vi "2_AdvancedDemo_MHHisto.vi"() -> ()   [LabVIEW 2010]
uses:
  Types/MH_UIThread_Cmds.ctl
  _lib/PQ/MultiHarp/MH_InitInfo.ctl
  Types/MH_UIThread_Data.ctl
  Types/MH_InputChannel.ctl
  _lib/PQ/MultiHarp/MH_RefSource.ctl
  _lib/PQ/MultiHarp/mhlib_x86_x64_UIThread.llb/MH_DllPath_global.vi
  <vilib>/Utility/error.llb/DialogType.ctl
  _lib/PQ/MultiHarp/MH_LibVersion_global.vi
  _lib/PQ/MultiHarp/MH_MeasMode.ctl
  Types/MH_SetInpChanData.ctl
  Types/MH_SetInpChanCmds.ctl
panel:
  in  "Settings":bool=TRUE
  in  "Run continuously":bool=TRUE caption="Conti."
  in  "Start":bool
  in  "Scale":bool
  out "CountRates":i32[](graph)
  in  "AllChannels":T1={"Enable"=TRUE, "Offset"=0, "Level"=-100, "Edge"=0, "DeadTime"=1000, "UseDeadTime"=FALSE, "SetEnableAllChan"=TRUE, "SetEdgeAllChan"=TRUE, "SetLevelAllChan"=TRUE, "SetOffsetAllChan"=TRUE, "SetUseDTAllChan"=TRUE, "SetDeadTAllChan"=TRUE} {"DeadTime" min=800 max=160000 step=1; "Edge" items=["falling", "rising"]; "Offset" min=-100000 max=100000 step=5; "Level" min=-1200 max=1200 step=1}
  in  "HistoLength":i32(ring)=6 caption="Num Bins" items=["1024", "2048", "4096", "8192", "16384", "32768", "65536"]
  in  "OvlLevel":u32=4294967295 caption="Ovl.Level" min=1 step=1
  in  "StopOvl.":bool=TRUE
  in  "AcqTime":i32=1000 caption="Acqu.           ms" min=1 max=360000 step=1
  in  "Binning":i32(ring) caption="Resol.            ps" items=["5", "10", "20", "40", "80", "160", "320", "640", "1280", "2560", "5120", "10240", "20480", "40960", "81920", "163840", "327680", "655360", "1310720", "2621440", "5242880", "10485760", "20971520", "41943040"]
  in  "HistoOffset":i32 caption="Offset            ns" min=0 max=100000000 step=1
  out "HistoGraph":T2(graph)={0.0, "Resolution"=0.005, "Histogram"=array64x1024[65536 elements]}
  in  "SyncDeadTime":i32=1000 caption="Dead T.   ps" min=800 max=160000 step=1
  in  "UseDeadTime":bool caption="Use DT."
  in  "SyncEdge":i32(ring) caption="Edge" items=["falling", "rising"]
  in  "SyncDivider":i32(ring) caption="Divider" items=["1", "2", "4", "8", "16"]
  in  "SyncOffset":i32 caption="Offset      ps" min=-100000 max=100000 step=5
  in  "SyncLevel":i32=-100 caption="Level      mV" min=-1200 max=1200 step=1
  in  "Channels":T3[](array[typedef])=[{"Name"="Inp.Chan 1", "Enable"=TRUE, "Edge"=0, "Level"=-100, "Offset"=0, "UseDeadTime"=FALSE, "DeadTime"=1000}, {"Name"="Inp.Chan 2", "Enable"=TRUE, "Edge"=0, "Level"=-100, "Offset"=0, "UseDeadTime"=FALSE, "DeadTime"=1000}, {"Name"="Inp.Chan 3", "Enable"=TRUE, "Edge"=0, "Level"=-100, "Offset"=0, "UseDeadTime"=FALSE, "DeadTime"=1000}, {"Name"="Inp.Chan 4", "Enable"=TRUE, "Edge"=0, "Level"=-100, "Offset"=0, "UseDeadTime"=FALSE, "DeadTime"=1000}, {"Name"="Inp.Chan 5", "Enable"=TRUE, "Edge"=0, "Level"=-100, "Offset"=0, "UseDeadTime"=FALSE, "DeadTime"=1000}, {"Name"="Inp.Chan 6", "Enable"=TRUE, "Edge"=0, "Level"=-100, "Offset"=0, "UseDeadTime"=FALSE, "DeadTime"=1000}, {"Name"="Inp.Chan 7", "Enable"=TRUE, "Edge"=0, "Level"=-100, "Offset"=0, "UseDeadTime"=FALSE, "DeadTime"=1000}, {"Name"="Inp.Chan 8", "Enable"=TRUE, "Edge"=0, "Level"=-100, "Offset"=0, "UseDeadTime"=FALSE, "DeadTime"=1000}, {"Name"="Inp.Chan 9", "Enable"=TRUE, "Edge"=0, "Level"=-100, "Offset"=0, "UseDeadTime"=FALSE, "DeadTime"=1000}, {"Name"="Inp.Chan 10", "Enable"=TRUE, "Edge"=0, "Level"=-100, "Offset"=0, "UseDeadTime"=FALSE, "DeadTime"=1000}, {"Name"="Inp.Chan 11", "Enable"=TRUE, "Edge"=0, "Level"=-100, "Offset"=0, "UseDeadTime"=FALSE, "DeadTime"=1000}, {"Name"="Inp.Chan 12", "Enable"=TRUE, "Edge"=0, "Level"=-100, "Offset"=0, "UseDeadTime"=FALSE, "DeadTime"=1000}, {"Name"="Inp.Chan 13", "Enable"=TRUE, "Edge"=0, "Level"=-100, "Offset"=0, "UseDeadTime"=FALSE, "DeadTime"=1000}, {"Name"="Inp.Chan 14", "Enable"=TRUE, "Edge"=0, "Level"=-100, "Offset"=0, "UseDeadTime"=FALSE, "DeadTime"=1000}, {"Name"="Inp.Chan 15", "Enable"=TRUE, "Edge"=0, "Level"=-100, "Offset"=0, "UseDeadTime"=FALSE, "DeadTime"=1000}, {"Name"="Inp.Chan 16", "Enable"=TRUE, "Edge"=0, "Level"=-100, "Offset"=0, "UseDeadTime"=FALSE, "DeadTime"=1000}, {"Name"="Inp.Chan 17", "Enable"=TRUE, "Edge"=0, "Level"=-100, "Offset"=0, "UseDeadTime"=FALSE, "DeadTime"=1000}, {"Name"="Inp.Chan 18", "Enable"=TRUE, "Edge"=0, "Level"=-100, "Offset"=0, "UseDeadTime"=FALSE, "DeadTime"=1000}, {"Name"="Inp.Chan 19", "Enable"=TRUE, "Edge"=0, "Level"=-100, "Offset"=0, "UseDeadTime"=FALSE, "DeadTime"=1000}, {"Name"="Inp.Chan 20", "Enable"=TRUE, "Edge"=0, "Level"=-100, "Offset"=0, "UseDeadTime"=FALSE, "DeadTime"=1000}, {"Name"="Inp.Chan 21", "Enable"=TRUE, "Edge"=0, "Level"=-100, "Offset"=0, "UseDeadTime"=FALSE, "DeadTime"=1000}, {"Name"="Inp.Chan 22", "Enable"=TRUE, "Edge"=0, "Level"=-100, "Offset"=0, "UseDeadTime"=FALSE, "DeadTime"=1000}, {"Name"="Inp.Chan 23", "Enable"=TRUE, "Edge"=0, "Level"=-100, "Offset"=0, "UseDeadTime"=FALSE, "DeadTime"=1000}, {"Name"="Inp.Chan 24", "Enable"=TRUE, "Edge"=0, "Level"=-100, "Offset"=0, "UseDeadTime"=FALSE, "DeadTime"=1000}, {"Name"="Inp.Chan 25", "Enable"=TRUE, "Edge"=0, "Level"=-100, "Offset"=0, "UseDeadTime"=FALSE, "DeadTime"=1000}, {"Name"="Inp.Chan 26", "Enable"=TRUE, "Edge"=0, "Level"=-100, "Offset"=0, "UseDeadTime"=FALSE, "DeadTime"=1000}, {"Name"="Inp.Chan 27", "Enable"=TRUE, "Edge"=0, "Level"=-100, "Offset"=0, "UseDeadTime"=FALSE, "DeadTime"=1000}, {"Name"="Inp.Chan 28", "Enable"=TRUE, "Edge"=0, "Level"=-100, "Offset"=0, "UseDeadTime"=FALSE, "DeadTime"=1000}, {"Name"="Inp.Chan 29", "Enable"=TRUE, "Edge"=0, "Level"=-100, "Offset"=0, "UseDeadTime"=FALSE, "DeadTime"=1000}, {"Name"="Inp.Chan 30", "Enable"=TRUE, "Edge"=0, "Level"=-100, "Offset"=0, "UseDeadTime"=FALSE, "DeadTime"=1000}, {"Name"="Inp.Chan 31", "Enable"=TRUE, "Edge"=0, "Level"=-100, "Offset"=0, "UseDeadTime"=FALSE, "DeadTime"=1000}, {"Name"="Inp.Chan 32", "Enable"=TRUE, "Edge"=0, "Level"=-100, "Offset"=0, "UseDeadTime"=FALSE, "DeadTime"=1000}, {"Name"="Inp.Chan 33", "Enable"=TRUE, "Edge"=0, "Level"=-100, "Offset"=0, "UseDeadTime"=FALSE, "DeadTime"=1000}, {"Name"="Inp.Chan 34", "Enable"=TRUE, "Edge"=0, "Level"=-100, "Offset"=0, "UseDeadTime"=FALSE, "DeadTime"=1000}, {"Name"="Inp.Chan 35", "Enable"=TRUE, "Edge"=0, "Level"=-100, "Offset"=0, "UseDeadTime"=FALSE, "DeadTime"=1000}, {"Name"="Inp.Chan 36", "Enable"=TRUE, "Edge"=0, "Level"=-100, "Offset"=0, "UseDeadTime"=FALSE, "DeadTime"=1000}, {"Name"="Inp.Chan 37", "Enable"=TRUE, "Edge"=0, "Level"=-100, "Offset"=0, "UseDeadTime"=FALSE, "DeadTime"=1000}, {"Name"="Inp.Chan 38", "Enable"=TRUE, "Edge"=0, "Level"=-100, "Offset"=0, "UseDeadTime"=FALSE, "DeadTime"=1000}, {"Name"="Inp.Chan 39", "Enable"=TRUE, "Edge"=0, "Level"=-100, "Offset"=0, "UseDeadTime"=FALSE, "DeadTime"=1000}, {"Name"="Inp.Chan 40", "Enable"=TRUE, "Edge"=0, "Level"=-100, "Offset"=0, "UseDeadTime"=FALSE, "DeadTime"=1000}, {"Name"="Inp.Chan 41", "Enable"=TRUE, "Edge"=0, "Level"=-100, "Offset"=0, "UseDeadTime"=FALSE, "DeadTime"=1000}, {"Name"="Inp.Chan 42", "Enable"=TRUE, "Edge"=0, "Level"=-100, "Offset"=0, "UseDeadTime"=FALSE, "DeadTime"=1000}, {"Name"="Inp.Chan 43", "Enable"=TRUE, "Edge"=0, "Level"=-100, "Offset"=0, "UseDeadTime"=FALSE, "DeadTime"=1000}, {"Name"="Inp.Chan 44", "Enable"=TRUE, "Edge"=0, "Level"=-100, "Offset"=0, "UseDeadTime"=FALSE, "DeadTime"=1000}, {"Name"="Inp.Chan 45", "Enable"=TRUE, "Edge"=0, "Level"=-100, "Offset"=0, "UseDeadTime"=FALSE, "DeadTime"=1000}, {"Name"="Inp.Chan 46", "Enable"=TRUE, "Edge"=0, "Level"=-100, "Offset"=0, "UseDeadTime"=FALSE, "DeadTime"=1000}, {"Name"="Inp.Chan 47", "Enable"=TRUE, "Edge"=0, "Level"=-100, "Offset"=0, "UseDeadTime"=FALSE, "DeadTime"=1000}, {"Name"="Inp.Chan 48", "Enable"=TRUE, "Edge"=0, "Level"=-100, "Offset"=0, "UseDeadTime"=FALSE, "DeadTime"=1000}, {"Name"="Inp.Chan 49", "Enable"=TRUE, "Edge"=0, "Level"=-100, "Offset"=0, "UseDeadTime"=FALSE, "DeadTime"=1000}, {"Name"="Inp.Chan 50", "Enable"=TRUE, "Edge"=0, "Level"=-100, "Offset"=0, "UseDeadTime"=FALSE, "DeadTime"=1000}, {"Name"="Inp.Chan 51", "Enable"=TRUE, "Edge"=0, "Level"=-100, "Offset"=0, "UseDeadTime"=FALSE, "DeadTime"=1000}, {"Name"="Inp.Chan 52", "Enable"=TRUE, "Edge"=0, "Level"=-100, "Offset"=0, "UseDeadTime"=FALSE, "DeadTime"=1000}, {"Name"="Inp.Chan 53", "Enable"=TRUE, "Edge"=0, "Level"=-100, "Offset"=0, "UseDeadTime"=FALSE, "DeadTime"=1000}, {"Name"="Inp.Chan 54", "Enable"=TRUE, "Edge"=0, "Level"=-100, "Offset"=0, "UseDeadTime"=FALSE, "DeadTime"=1000}, {"Name"="Inp.Chan 55", "Enable"=TRUE, "Edge"=0, "Level"=-100, "Offset"=0, "UseDeadTime"=FALSE, "DeadTime"=1000}, {"Name"="Inp.Chan 56", "Enable"=TRUE, "Edge"=0, "Level"=-100, "Offset"=0, "UseDeadTime"=FALSE, "DeadTime"=1000}, {"Name"="Inp.Chan 57", "Enable"=TRUE, "Edge"=0, "Level"=-100, "Offset"=0, "UseDeadTime"=FALSE, "DeadTime"=1000}, {"Name"="Inp.Chan 58", "Enable"=TRUE, "Edge"=0, "Level"=-100, "Offset"=0, "UseDeadTime"=FALSE, "DeadTime"=1000}, {"Name"="Inp.Chan 59", "Enable"=TRUE, "Edge"=0, "Level"=-100, "Offset"=0, "UseDeadTime"=FALSE, "DeadTime"=1000}, {"Name"="Inp.Chan 60", "Enable"=TRUE, "Edge"=0, "Level"=-100, "Offset"=0, "UseDeadTime"=FALSE, "DeadTime"=1000}, {"Name"="Inp.Chan 61", "Enable"=TRUE, "Edge"=0, "Level"=-100, "Offset"=0, "UseDeadTime"=FALSE, "DeadTime"=1000}, {"Name"="Inp.Chan 62", "Enable"=TRUE, "Edge"=0, "Level"=-100, "Offset"=0, "UseDeadTime"=FALSE, "DeadTime"=1000}, {"Name"="Inp.Chan 63", "Enable"=TRUE, "Edge"=0, "Level"=-100, "Offset"=0, "UseDeadTime"=FALSE, "DeadTime"=1000}, {"Name"="Inp.Chan 64", "Enable"=TRUE, "Edge"=0, "Level"=-100, "Offset"=0, "UseDeadTime"=FALSE, "DeadTime"=1000}] {"DeadTime" min=800 max=160000 step=1; "Edge" items=["falling", "rising"]; "Offset" min=-100000 max=100000 step=5; "Level" min=-1200 max=1200 step=1}
  out "SyncRate":string="Sync Rate: 0 cps\n"
  out "OverFlow":bool caption="Overflow:"
  out "Status":string="Initialized!"
  # "Acquisition"
  # "All Channels"
  # "Sync"
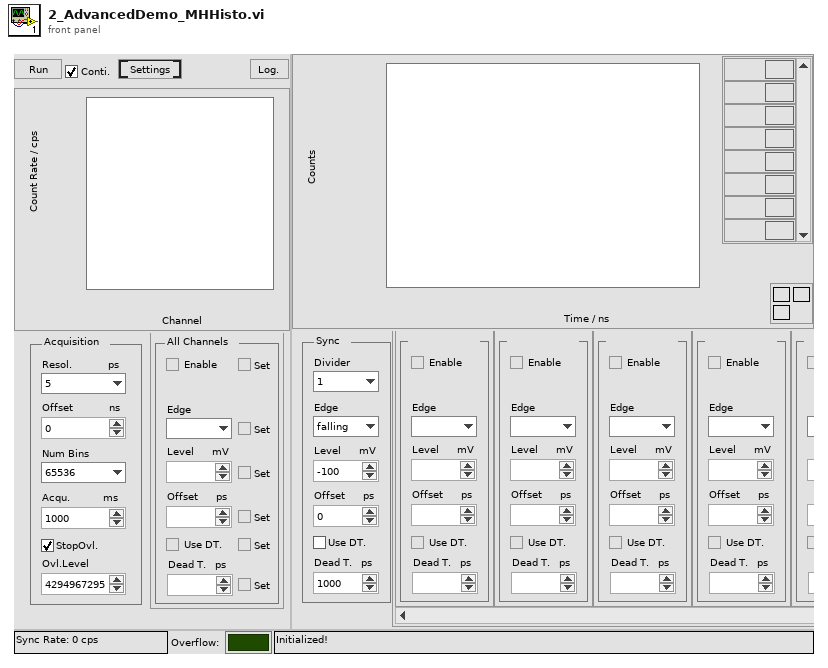
[diagram p1: front panel]
types:
  T1 = cluster{"Enable":bool, "Offset":i32, "Level":i32, "Edge":i32, "DeadTime":i32, "UseDeadTime":bool, "SetEnableAllChan":bool, "SetEdgeAllChan":bool, "SetLevelAllChan":bool, "SetOffsetAllChan":bool, "SetUseDTAllChan":bool, "SetDeadTAllChan":bool}
  T2 = cluster{dbl, "Resolution":dbl, "Histogram":u32[][]}
  T3 = typedef "MH_InputChannel.ctl" = cluster{"Name":string, "Enable":bool, "Edge":i32, "Level":i32, "Offset":i32, "UseDeadTime":bool, "DeadTime":i32}
  T4 = typedef "MH_UIThread_Data.ctl" = cluster{"Init Info":T5, "DevIdx":i32, "SyncDivider":i32, "SyncOffset":i32, "SyncLevel":i32, "Channels":T3[], "CurrentChannels":i32[], "AcqTime":i32, "Binning":i32, "HistoOffset":i32, "HistoLen":i32, "StopOvl.":bool, "OvlLevel":u32, "SyncEdge":i32, "StartMeas":bool, "HistoLength":i32, "Resolution":dbl, "Run cont.":bool, "Status":string, "SyncRate":i32, "BitShift":i32, "HistoAcqTime":dbl, "SyncRateStart":i32, "UseDeadTime":bool, "SyncDeadTime":i32, "SetInpChan":T6[]}
  T5 = typedef "MH_InitInfo.ctl" = cluster{"Library Version":string, "Serial No.":string, "Model":string, "Partnum":string, "Version":string, "features":i32, "nchannels":i32, "Base Resolution":dbl, "Bin Steps":i32}
  T6 = typedef "MH_SetInpChanData.ctl" = cluster{"Channel":i32, "Cmds":T7[], "Changed":cluster{"Name":bool, "Enable":bool, "Edge":bool, "Level":bool, "Offset":bool, "UseDeadTime":bool, "DeadTime":bool}}
  T7 = typedef "MH_SetInpChanCmds.ctl" = enum16{"SetInpChanEnable", "SetInpChanOffset", "SetInpChanDeadTime", "SetInpChanTrg"}
  T8 = typedef "MH_UIThread_Cmds.ctl" = enum16{"Idle", "Init", "SetInpChan", "SetSyncDivider", "SetSyncTrg", "SetSyncOffset", "SetSyncDeadTime", "SetBinning", "SetHistoOffset", "SetHistoLen", "SetStopOvl", "SetBitShift", "SetHistoAcqTime", "GetRates", "GetAllRates", "StartMeas", "StopMeas", "AbortMeas", "GetResolution", "GetHistos", "GetAllHistos", "ReadFiFo", "WriteStatus", "Resize", "EnableControls", "DisableControls", "Error", "Exit"}
  T9 = enum8{"Enabled", "Disabled", "Disabled and Grayed Out"}
  T10 = cluster{"[0]":bool, "[1]":bool, "[2]":bool, "[3]":bool, "[4]":bool, "[5]":bool}
  T11 = typedef "MH_MeasMode.ctl" = i32
  T12 = typedef "MH_RefSource.ctl" = enum16{"INTERNAL", "EXTERNAL_10MHZ", "WR_MASTER_GENERIC", "WR_SLAVE_GENERIC", "WR_GRANDM_GENERIC", "EXTN_GPS_PPS", "EXTN_GPS_PPS_UART", "WR_MASTER_MHARP", "WR_SLAVE_MHARP", "WR_GRANDM_MHARP"}
  T13 = cluster{dbl, "Resolution":dbl, "Histograms":u32[][]}
  T14 = typedef "DialogType.ctl" = u16
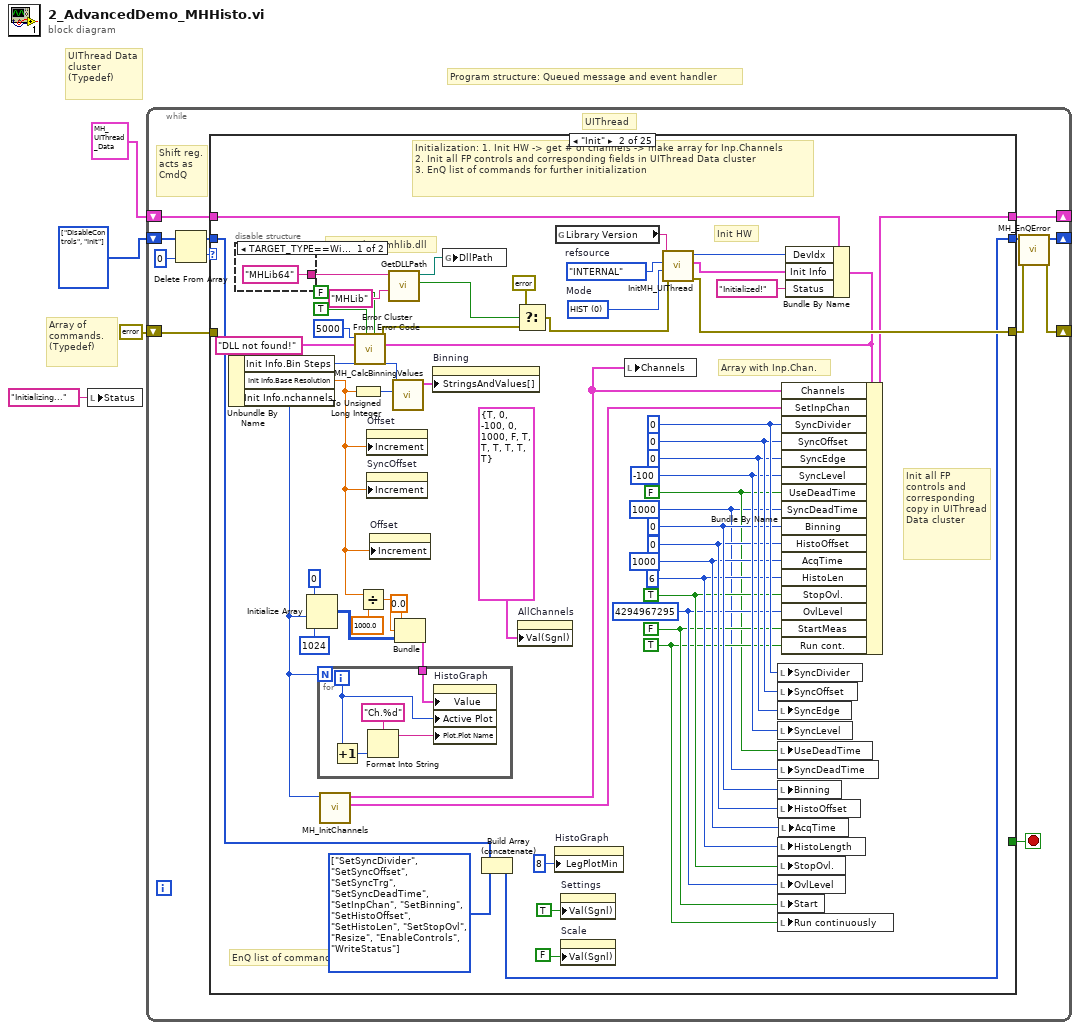
[diagram p0: block diagram]
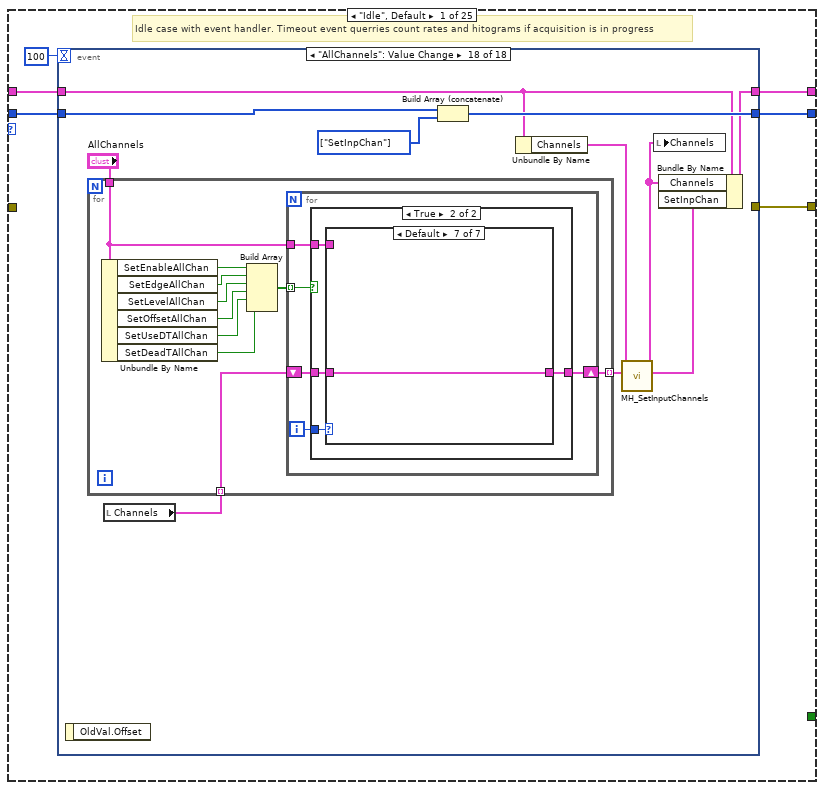
[diagram p2: hidden frame]
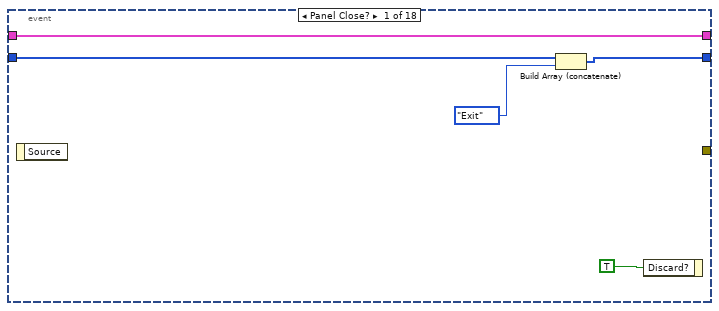
[diagram p3: hidden frame]
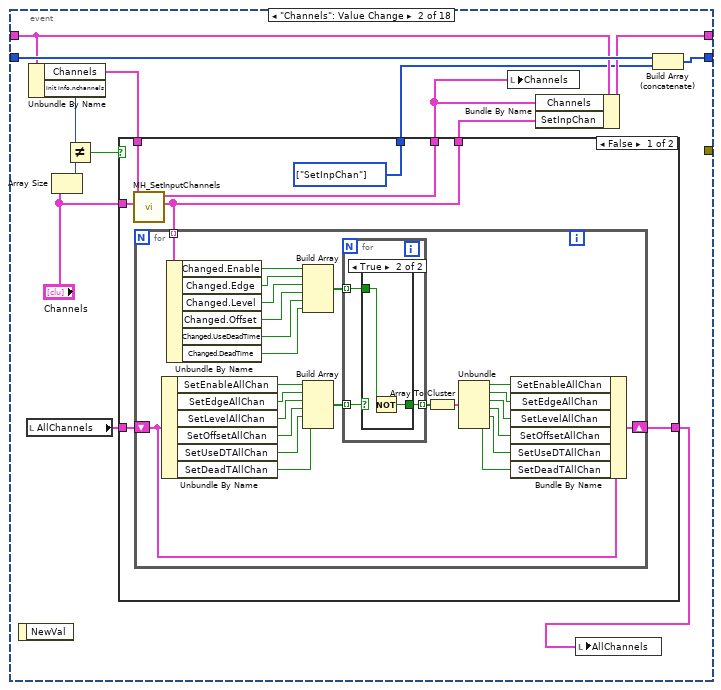
[diagram p4: hidden frame]
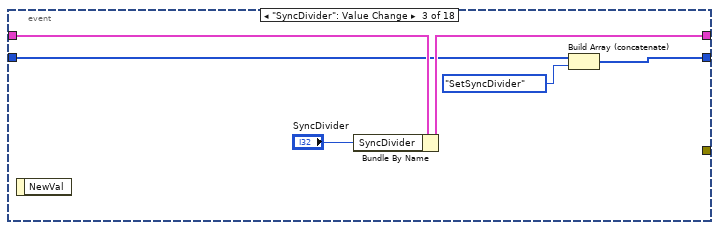
[diagram p7: hidden frame]
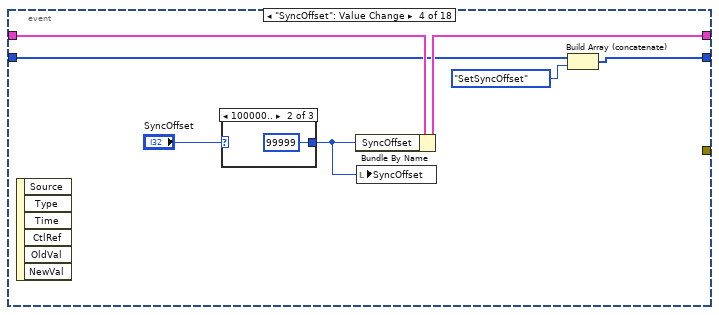
[diagram p8: hidden frame]
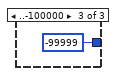
[diagram p10: hidden frame]
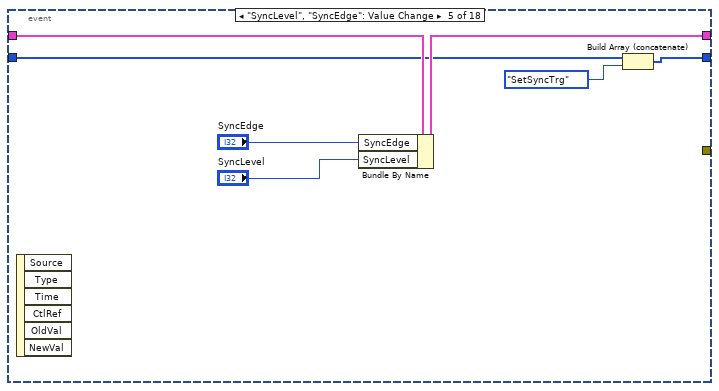
[diagram p11: hidden frame]
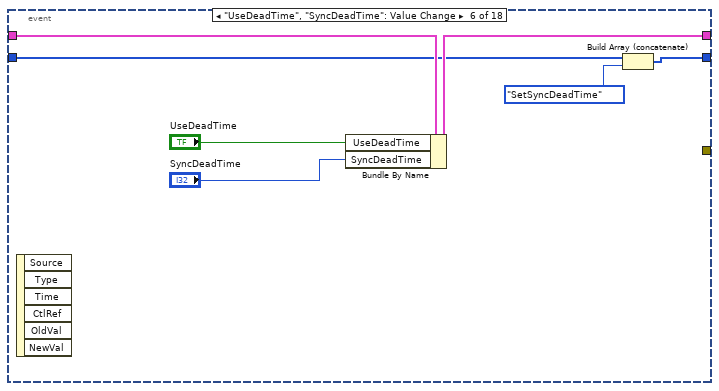
[diagram p12: hidden frame]
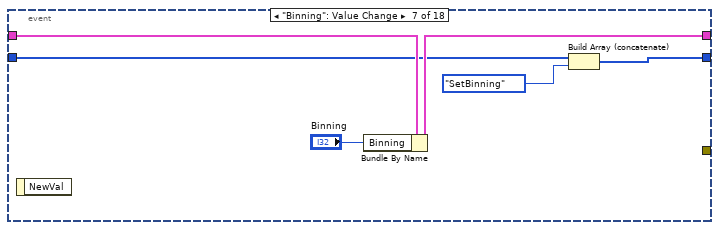
[diagram p13: hidden frame]
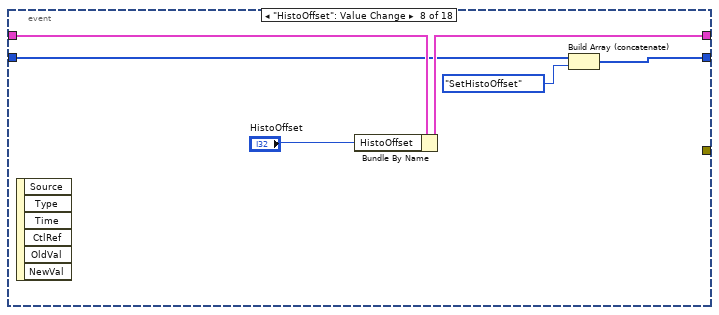
[diagram p14: hidden frame]
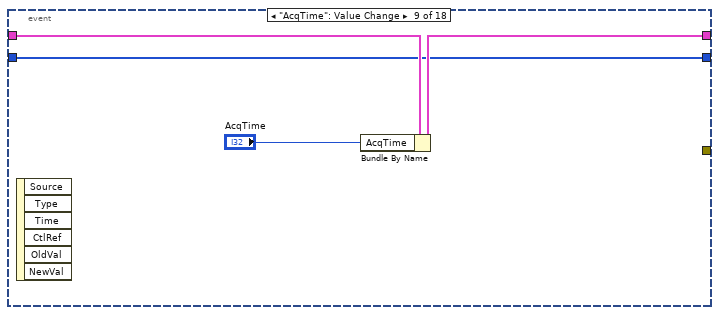
[diagram p15: hidden frame]
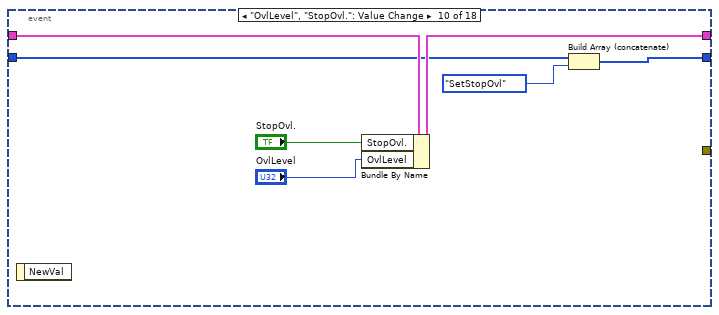
[diagram p16: hidden frame]
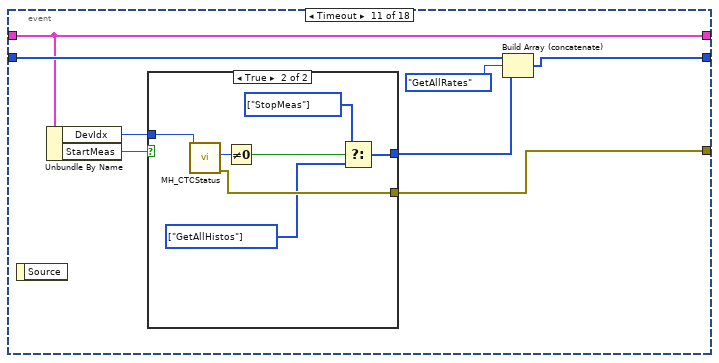
[diagram p17: hidden frame]
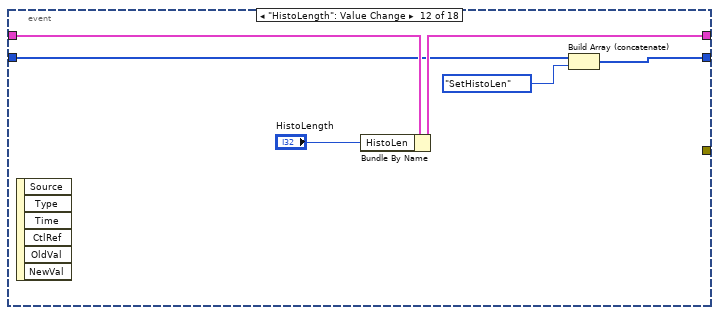
[diagram p19: hidden frame]
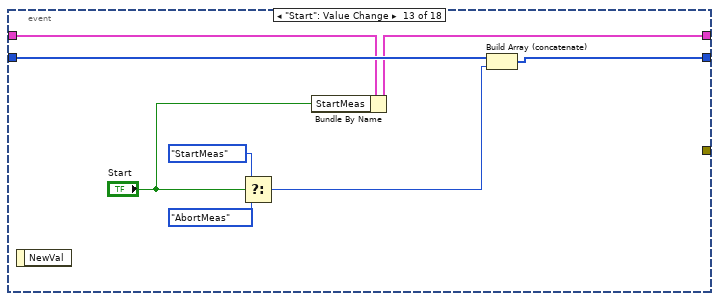
[diagram p20: hidden frame]
diagram:
  w3 = T8[] [enum."DisableControls", enum."Init"] items=["Idle", "Init", "SetInpChan", "SetSyncDivider", "SetSyncTrg", "SetSyncOffset", "SetSyncDeadTime", "SetBinning", "SetHistoOffset", "SetHistoLen", "SetStopOvl", "SetBitShift", "SetHistoAcqTime", "GetRates", "GetAllRates", "StartMeas", "StopMeas", "AbortMeas", "GetResolution", "GetHistos", "GetAllHistos", "ReadFiFo", "WriteStatus", "Resize", "EnableControls", "DisableControls", "Error", "Exit"]
  # "Array of commands.\n(Typedef)"
  # "Program structure: Queued message and event handler"
  # "UIThread Data cluster\n(Typedef)"
  n1 = local write "Status"("Initializing..." ("Status")) -> ()
  n2 = while {
    shift-right: [w5] -> _
    shift-left: w3 -> [w12]
    shift-right: [w15] -> _
    shift-left: T4 {"Init Info"={"Library Version"="", "Serial No."="", "Model"="", "Partnum"="", "Version"="", "features"=0, "nchannels"=0, "Base Resolution"=0.0, "Bin Steps"=0}, "DevIdx"=0, "SyncDivider"=1, "SyncOffset"=0, "SyncLevel"=50, "Channels"=[], "CurrentChannels"=[], "AcqTime"=1, "Binning"=1, "HistoOffset"=1, "HistoLen"=1024, "StopOvl."=FALSE, "OvlLevel"=1024, "SyncEdge"=10, "StartMeas"=FALSE, "HistoLength"=0, "Resolution"=0.0, "Run cont."=FALSE, "Status"="", "SyncRate"=0, "BitShift"=0, "HistoAcqTime"=0.0, "SyncRateStart"=0, "UseDeadTime"=FALSE, "SyncDeadTime"=800, "SetInpChan"=[]} -> [w14]
    shift-right: [w7] -> _
    shift-left: errorcluster {"status"=FALSE, "code"=0, "source"=""} ("error IO") -> [w13]
    stop <- w16 stop-if-true
    # "Shift reg.\nacts as\nCmdQ"
    # "UIThread"
    n3 = Delete From Array(array=w12, index=0) -> (deleted portion=w10:T8, array with subset deleted=w9:T8[])  [unwired: 1 in]
    n4 = case shown="\"Init\"" w10 {
      tunnel: [w22 w305 w324 w386 w395 w407 w413 w420 w428 w436 w441 w452 w463 w478 w486 w500 w514 w539 w571 w595 w608 w615 w627 w633 w637] -> w6
      tunnel: [_ _ _ _ _ _ _ _ _ _ _ _ _ _ _ _ _ _ _ _ _ _ _ _ TRUE] -> w16
      tunnel: [w21 w285 w325 w388 w396 w408 w417 w424 w429 w431 w442 w451 w462 w484 w489 w503 w510 w538 w570 w594 w596 w614 w626 w634 w640] -> w15
      tunnel: w14 -> [w20 w290 w325 w388 w396 w408 w417 w424 w429 w432 w442 w451 w462 w484 w490 w504 w511 w538 w570 w594 w596 w614 w626 w634 w640]
      tunnel: [w17 w308 w322 w384 w394 w406 w416 w423 w427 w435 w440 w445 w461 w483 w492 w506 w512 w536 w566 _ _ _ _ _ w638] -> w8
      tunnel: w13 -> [_ _ _ _ _ _ _ _ _ _ _ _ _ _ _ _ _ _ _ _ _ _ _ w635 _]
      tunnel: w9 -> [w19 w307 w324 w386 w395 w407 w413 w419 w428 w436 w441 w452 w463 w479 w487 w501 w514 w539 w571 w595 w608 w615 w627 _ w637]
      frame "Idle", Default {
        # "Idle case with event handler. Timeout event querries count rates and hitograms if acquisition is in progress"
        n5 = event shown="[17] \"AllChannels\": Value Change" {
          selector: _ -> [_ _ _ _ _ _ _ _ _ _ _ _ _ _ _ _ _ _]
          dyn-events: _ -> [_ _ _ _ _ _ _ _ _ _ _ _ _ _ _ _ _ _]
          timeout: 100 -> [_ _ _ _ _ _ _ _ _ _ _ _ _ _ _ _ _ _]
          tunnel: [w23 w40 w82 w90 w99 w107 w113 w119 w124 w130 w140 w151 w159 w167 w173 w181 w191 w204] -> w22
          tunnel: [w26 w33 w86 w93 w103 w110 w116 w122 w126 w133 w139 w154 w157 w165 w172 w180 w194 w198] -> w21
          tunnel: w20 -> [w26 w35 w87 w94 w104 w111 w117 w123 w127 w134 w139 w155 w158 w166 w172 w180 w194 w199]
          tunnel: w19 -> [w25 w41 w84 w92 w101 w109 w115 w121 w124 w132 w142 w153 w161 w167 w173 w181 w192 w205]
          tunnel: [_ _ _ _ _ _ _ _ _ _ w135 _ _ _ _ _ _ _] -> w17
          event Panel Close? {
            n6 = event-data() -> ()  [unwired: 1 in, 1 out]
            n7 = Build Array (concatenate)(w25, MH_UIThread_Cmds."Exit") -> (w23:T8[])
            n8 = event-data("Discard?"=TRUE) -> ()  [unwired: 1 in, 1 out]
          }
          event "Channels": Value Change {
            n9 = event-data() -> ()  [unwired: 1 in, 1 out]
            n10 = local read "AllChannels"() -> (w29:T1)
            n11 = Unbundle By Name(w35) -> ("Channels"=w36:T3[], "Init Info.nchannels"=w39:i32)
            n12 = Array Size(array="Channels") -> (size(s)=w38:i32)
            n13 = Not Equal?(x=w39, y=w38) -> (x != y?=w37:bool)
            n14 = case shown="False" w37 {
              tunnel: "Channels" -> [w47 _]
              tunnel: [w46 w81] -> w34
              tunnel: w36 -> [w48 w81]
              tunnel: [w44 _] -> w32
              tunnel: [w45 _] -> w30
              tunnel: w29 -> [w43 w80]
              tunnel: [w42 w80] -> w28
              frame False {
                w45 = T8[] [enum."SetInpChan"] items=["Idle", "Init", "SetInpChan", "SetSyncDivider", "SetSyncTrg", "SetSyncOffset", "SetSyncDeadTime", "SetBinning", "SetHistoOffset", "SetHistoLen", "SetStopOvl", "SetBitShift", "SetHistoAcqTime", "GetRates", "GetAllRates", "StartMeas", "StopMeas", "AbortMeas", "GetResolution", "GetHistos", "GetAllHistos", "ReadFiFo", "WriteStatus", "Resize", "EnableControls", "DisableControls", "Error", "Exit"] ("array")
                n15 = call "MH_SetInputChannels.vi"("Channels new"=w47, "Channels old"=w48) -> ("SetInpChan"=w44:T6[], "Channels"=w46:T3[])  [unwired: 8 in]
                n16 = for {
                  tunnel: w44 -> [w73] mode=indexing
                  shift-right: [w55] -> w42
                  shift-left: w43 -> [w57]
                  n17 = Unbundle By Name(w57) -> ("SetEnableAllChan"=w66:bool, "SetEdgeAllChan"=w65:bool, "SetLevelAllChan"=w64:bool, "SetOffsetAllChan"=w63:bool, "SetUseDTAllChan"=w62:bool, "SetDeadTAllChan"=w61:bool)
                  n18 = Unbundle By Name(w73) -> ("Changed.Enable"=w72:bool, "Changed.Edge"=w71:bool, "Changed.Level"=w70:bool, "Changed.Offset"=w69:bool, "Changed.UseDeadTime"=w68:bool, "Changed.DeadTime"=w67:bool)
                  n19 = Build Array(w72, w71, w70, w69, w68, w67) -> (w59:bool[])
                  n20 = Build Array(w66, w65, w64, w63, w62, w61) -> (w60:bool[])
                  n21 = for {
                    tunnel: w60 -> [w76] mode=indexing
                    tunnel: w59 -> [w74] mode=indexing
                    tunnel: [w75] -> w58 mode=indexing
                    n22 = case shown="True" w76 {
                      selector: w76 -> [w77 _]
                      tunnel: [w77 w78] -> w75
                      tunnel: w74 -> [_ w79]
                      frame False {
                      }
                      frame True {
                        n23 = Not(x=w79) -> (.not. x?=w78:bool)
                      }
                    }
                  }
                  n24 = Array To Cluster(array=w58) -> (cluster=w56:T10)
                  n25 = Unbundle(w56) -> ("[0]"=w54:bool, "[1]"=w53:bool, "[2]"=w52:bool, "[3]"=w51:bool, "[4]"=w50:bool, "[5]"=w49:bool)
                  n26 = Bundle By Name(cluster=w57, "SetEnableAllChan"=w54, "SetEdgeAllChan"=w53, "SetLevelAllChan"=w52, "SetOffsetAllChan"=w51, "SetUseDTAllChan"=w50, "SetDeadTAllChan"=w49) -> (w55:T1)
                }
              }
              frame True {
              }
            }
            n27 = local write "Channels"(w34) -> ()
            n28 = Bundle By Name(cluster=w35, "Channels"=w34, "SetInpChan"=w32) -> (w33:T4)
            n29 = local write "AllChannels"(w28) -> ()
            n30 = Build Array (concatenate)(w41, w30) -> (w40:T8[])
          }
          event "SyncDivider": Value Change {
            n31 = event-data() -> ()  [unwired: 1 in, 1 out]
            n32 = Bundle By Name(cluster=w87, "SyncDivider"="SyncDivider") -> (w86:T4)
            n33 = Build Array (concatenate)(w84, MH_UIThread_Cmds."SetSyncDivider") -> (w82:T8[])
          }
          event "SyncOffset": Value Change {
            n34 = event-data() -> ()  [unwired: 1 in, 6 out]
            n35 = case shown="100000.." "SyncOffset" {
              selector: "SyncOffset" -> [w95 _ _]
              tunnel: [w95 99999 ("SyncOffset") -99999 ("SyncOffset")] -> w88
              frame Default {
              }
              frame 100000.. {
              }
              frame ..-100000 {
              }
            }
            n36 = Bundle By Name(cluster=w94, "SyncOffset"=w88) -> (w93:T4)
            n37 = local write "SyncOffset"(w88) -> ()
            n38 = Build Array (concatenate)(w92, MH_UIThread_Cmds."SetSyncOffset") -> (w90:T8[])
          }
          event "SyncLevel", "SyncEdge": Value Change {
            n39 = event-data() -> ()  [unwired: 1 in, 6 out]
            n40 = Bundle By Name(cluster=w104, "SyncEdge"="SyncEdge", "SyncLevel"="SyncLevel") -> (w103:T4)
            n41 = Build Array (concatenate)(w101, MH_UIThread_Cmds."SetSyncTrg") -> (w99:T8[])
          }
          event "UseDeadTime", "SyncDeadTime": Value Change {
            n42 = event-data() -> ()  [unwired: 1 in, 6 out]
            n43 = Bundle By Name(cluster=w111, "UseDeadTime"="UseDeadTime", "SyncDeadTime"="SyncDeadTime") -> (w110:T4)
            n44 = Build Array (concatenate)(w109, MH_UIThread_Cmds."SetSyncDeadTime") -> (w107:T8[])
          }
          event "Binning": Value Change {
            n45 = event-data() -> ()  [unwired: 1 in, 1 out]
            n46 = Bundle By Name(cluster=w117, "Binning"="Binning") -> (w116:T4)
            n47 = Build Array (concatenate)(w115, MH_UIThread_Cmds."SetBinning") -> (w113:T8[])
          }
          event "HistoOffset": Value Change {
            n48 = event-data() -> ()  [unwired: 1 in, 6 out]
            n49 = Bundle By Name(cluster=w123, "HistoOffset"="HistoOffset") -> (w122:T4)
            n50 = Build Array (concatenate)(w121, MH_UIThread_Cmds."SetHistoOffset") -> (w119:T8[])
          }
          event "AcqTime": Value Change {
            n51 = event-data() -> ()  [unwired: 1 in, 6 out]
            n52 = Bundle By Name(cluster=w127, "AcqTime"="AcqTime") -> (w126:T4)
          }
          event "OvlLevel", "StopOvl.": Value Change {
            n53 = event-data() -> ()  [unwired: 1 in, 1 out]
            n54 = Bundle By Name(cluster=w134, "StopOvl."="StopOvl.", "OvlLevel"="OvlLevel") -> (w133:T4)
            n55 = Build Array (concatenate)(w132, MH_UIThread_Cmds."SetStopOvl") -> (w130:T8[])
          }
          event Timeout {
            n56 = event-data() -> ()  [unwired: 1 in, 1 out]
            n57 = Unbundle By Name(w139) -> ("DevIdx"=w137:i32, "StartMeas"=w138:bool)
            n58 = case shown="True" w138 {
              tunnel: w137 -> [_ w149]
              tunnel: [_ w147] -> w136
              tunnel: [_ w145] -> w135
              frame False {
              }
              frame True {
                w143 = T8[] [enum."GetAllHistos"] items=["Idle", "Init", "SetInpChan", "SetSyncDivider", "SetSyncTrg", "SetSyncOffset", "SetSyncDeadTime", "SetBinning", "SetHistoOffset", "SetHistoLen", "SetStopOvl", "SetBitShift", "SetHistoAcqTime", "GetRates", "GetAllRates", "StartMeas", "StopMeas", "AbortMeas", "GetResolution", "GetHistos", "GetAllHistos", "ReadFiFo", "WriteStatus", "Resize", "EnableControls", "DisableControls", "Error", "Exit"]
                w146 = T8[] [enum."StopMeas"] items=["Idle", "Init", "SetInpChan", "SetSyncDivider", "SetSyncTrg", "SetSyncOffset", "SetSyncDeadTime", "SetBinning", "SetHistoOffset", "SetHistoLen", "SetStopOvl", "SetBitShift", "SetHistoAcqTime", "GetRates", "GetAllRates", "StartMeas", "StopMeas", "AbortMeas", "GetResolution", "GetHistos", "GetAllHistos", "ReadFiFo", "WriteStatus", "Resize", "EnableControls", "DisableControls", "Error", "Exit"]
                n59 = call "MH_CTCStatus.vi"("devidx"=w149) -> ("error out"=w145:errorcluster, "ctcstatus"=w148:i32)  [unwired: 8 in, 1 out]
                n60 = Not Equal To 0?(x=w148) -> (x != 0?=w144:bool)
                n61 = Select(t=w146, s=w144, f=w143) -> (s? t:f=w147:T8[])
              }
            }
            n62 = Build Array (concatenate)(w142, MH_UIThread_Cmds."GetAllRates", w136) -> (w140:T8[])
          }
          event "HistoLength": Value Change {
            n63 = event-data() -> ()  [unwired: 1 in, 6 out]
            n64 = Bundle By Name(cluster=w155, "HistoLen"="HistoLength") -> (w154:T4)
            n65 = Build Array (concatenate)(w153, MH_UIThread_Cmds."SetHistoLen") -> (w151:T8[])
          }
          event "Start": Value Change {
            n66 = event-data() -> ()  [unwired: 1 in, 1 out]
            n67 = Select(t=MH_UIThread_Cmds."StartMeas", s="Start", f=MH_UIThread_Cmds."AbortMeas") -> (s? t:f=w160:T8)
            n68 = Bundle By Name(cluster=w158, "StartMeas"="Start") -> (w157:T4)
            n69 = Build Array (concatenate)(w161, w160) -> (w159:T8[])
          }
          event "Run continuously": Value Change {
            n70 = event-data() -> ()  [unwired: 1 in, 1 out]
            n71 = Bundle By Name(cluster=w166, "Run cont."="Run continuously") -> (w165:T4)
          }
          event "Scale": Value Change {
            n72 = event-data() -> ()  [unwired: 1 in, 1 out]
            n73 = Select(t=u8 0 ("Y Scale.Mapping Mode"), s="Scale", f=u8 1 ("Y Scale.Mapping Mode")) -> (s? t:f=w168:u8)
            n74 = property on="HistoGraph" class="WFGraph (strict)"("YScale.Mapping Mode"=w168) -> ()  [unwired: 2 in, 2 out]
          }
          event "Settings": Value Change {
            n75 = event-data() -> ()  [unwired: 1 in, 1 out]
            n76 = property on="Splitter" class="Splitter"() -> ("Position"=w179:i32)  [unwired: 2 in, 2 out]
            n77 = Select(t=300 ("PosT"), s="Settings", f=0 ("PosF")) -> (s? t:f=w176:i32)
            n78 = Subtract(x=w179, y=w176) -> (x-y=w175:i32)
            n79 = while {
              shift-right: [w190] -> _
              shift-left: w175 -> [w183]
              i -> [w189]
              stop <- w186 stop-if-true
              n80 = property on="Splitter 4" class="Splitter"("Position"=w183) -> (error out=w182:errorcluster)  [unwired: 2 in, 1 out]
              n81 = Greater Or Equal?(x=w189, y=10) -> (x >= y?=w187:bool)
              n82 = Decrement(x=w183) -> (x-1=w190:i32)
              n83 = Unbundle(w182) -> ("status"=w185:bool)  [unwired: 2 out]
              n84 = Not(x=w185) -> (.not. x?=w184:bool)
              n85 = Or(x=w184, y=w187) -> (x .or. y?=w186:bool)
            }
          }
          event Panel Resize {
            n86 = event-data() -> ()  [unwired: 1 in, 1 out]
            n87 = Build Array (concatenate)(w192, MH_UIThread_Cmds."Resize") -> (w191:T8[])
          }
          event "AllChannels": Value Change {
            w196 = T8[] [enum."SetInpChan"] items=["Idle", "Init", "SetInpChan", "SetSyncDivider", "SetSyncTrg", "SetSyncOffset", "SetSyncDeadTime", "SetBinning", "SetHistoOffset", "SetHistoLen", "SetStopOvl", "SetBitShift", "SetHistoAcqTime", "GetRates", "GetAllRates", "StartMeas", "StopMeas", "AbortMeas", "GetResolution", "GetHistos", "GetAllHistos", "ReadFiFo", "WriteStatus", "Resize", "EnableControls", "DisableControls", "Error", "Exit"] ("array")
            n88 = event-data() -> ()  [unwired: 1 in, 1 out]
            n89 = local read "Channels"() -> (w203:T3[])
            n90 = for {
              tunnel: w203 -> [w208] mode=indexing
              tunnel: "AllChannels" -> [w207]
              tunnel: [w206] -> w201 mode=indexing
              n91 = Unbundle By Name(w207) -> ("SetEnableAllChan"=w209:bool, "SetEdgeAllChan"=w210:bool, "SetLevelAllChan"=w211:bool, "SetOffsetAllChan"=w212:bool, "SetUseDTAllChan"=w213:bool, "SetDeadTAllChan"=w214:bool)
              n92 = Build Array(w209, w210, w211, w212, w213, w214) -> (w215:bool[])
              n93 = for {
                tunnel: w215 -> [w220] mode=indexing
                shift-right: [w217] -> w206
                shift-left: w208 -> [w218]
                tunnel: w207 -> [w216]
                i -> [w219]
                n94 = case shown="True" w220 {
                  tunnel: w219 -> [_ w225]
                  tunnel: w216 -> [_ w224]
                  tunnel: w218 -> [w221 w223]
                  tunnel: [w221 w222] -> w217
                  frame False {
                  }
                  frame True {
                    n95 = case shown="Default" w225 {
                      tunnel: w224 -> [w229 w233 w237 w242 w249 w253 _]
                      tunnel: w223 -> [w228 w232 w236 w241 w248 w252 w254]
                      tunnel: [w226 w230 w234 w240 w246 w250 w254] -> w222
                      frame 0 {
                        n96 = Unbundle By Name(w229) -> ("Enable"=w227:bool)
                        n97 = Bundle By Name(cluster=w228, "Enable"=w227) -> (w226:T3)
                      }
                      frame 1 {
                        n98 = Unbundle By Name(w233) -> ("Edge"=w231:i32)
                        n99 = Bundle By Name(cluster=w232, "Edge"=w231) -> (w230:T3)
                      }
                      frame 2 {
                        n100 = Unbundle By Name(w237) -> ("Level"=w235:i32)
                        n101 = Bundle By Name(cluster=w236, "Level"=w235) -> (w234:T3)
                      }
                      frame 3 {
                        n102 = Unbundle By Name(w242) -> ("Offset"=w239:i32)
                        n103 = case shown="100000.." w239 {
                          selector: w239 -> [w243 _ _]
                          tunnel: [w243 99999 ("SyncOffset") -99999 ("SyncOffset")] -> w238
                          frame Default {
                          }
                          frame 100000.. {
                          }
                          frame ..-100000 {
                          }
                        }
                        n104 = Bundle By Name(cluster=w241, "Offset"=w238) -> (w240:T3)
                      }
                      frame 4 {
                        n105 = Unbundle By Name(w249) -> ("UseDeadTime"=w247:bool)
                        n106 = Bundle By Name(cluster=w248, "UseDeadTime"=w247) -> (w246:T3)
                      }
                      frame 5 {
                        n107 = Unbundle By Name(w253) -> ("DeadTime"=w251:i32)
                        n108 = Bundle By Name(cluster=w252, "DeadTime"=w251) -> (w250:T3)
                      }
                      frame Default {
                      }
                    }
                  }
                }
              }
            }
            n109 = Build Array (concatenate)(w205, w196) -> (w204:T8[])
            n110 = Unbundle By Name(w199) -> ("Channels"=w200:T3[])
            n111 = call "MH_SetInputChannels.vi"("Channels new"=w201, "Channels old"=w200) -> ("SetInpChan"=w197:T6[], "Channels"=w195:T3[])  [unwired: 8 in]
            n112 = local write "Channels"(w195) -> ()
            n113 = Bundle By Name(cluster=w199, "Channels"=w195, "SetInpChan"=w197) -> (w198:T4)
          }
        }
      }
      frame "Init" {
        w266 = 1000 ("SyncDeadTime")
        w267 = FALSE ("UseDeadTime")
        w269 = T11 0 items=["HIST"=0, "T2"=2, "T3"=3]  # Mode
        w278 = MH_RefSource."INTERNAL"  # refsource
        w292 = TRUE ("Run cont.")
        w294 = FALSE ("StartMeas")
        w295 = u32 4294967295 ("OvlLevel")
        w296 = TRUE ("StopOvl.")
        w297 = 6 ("HistoLen")
        w298 = 1000 ("AcqTime")
        w299 = 0 ("HistoOffset")
        w300 = 0 ("Binning")
        w301 = -100 ("SyncLevel")
        w302 = 0 ("SyncZeroX")
        w303 = 0 ("SyncOffset")
        w304 = 0 ("SyncDivider")
        w306 = T8[] [enum."SetSyncDivider", enum."SetSyncOffset", enum."SetSyncTrg", enum."SetSyncDeadTime", enum."SetInpChan", enum."SetBinning", enum."SetHistoOffset", enum."SetHistoLen", enum."SetStopOvl", enum."Resize", enum."EnableControls", enum."WriteStatus"] items=["Idle", "Init", "SetInpChan", "SetSyncDivider", "SetSyncTrg", "SetSyncOffset", "SetSyncDeadTime", "SetBinning", "SetHistoOffset", "SetHistoLen", "SetStopOvl", "SetBitShift", "SetHistoAcqTime", "GetRates", "GetAllRates", "StartMeas", "StopMeas", "AbortMeas", "GetResolution", "GetHistos", "GetAllHistos", "ReadFiFo", "WriteStatus", "Resize", "EnableControls", "DisableControls", "Error", "Exit"]
        # "Init HW"
        # "Set path to mhlib.dll"
        # "Init all FP controls and corresponding copy in UIThread Data cluster"
        # "EnQ list of commands"
        # "Array with Inp.Chan."
        # "Initialization: 1. Init HW -> get # of channels -> make array for Inp.Channels\n2. Init all FP controls and corresponding fields in UIThread Data cluster\n3. EnQ list of commands for further initialization"
        n114 = disable-structure shown="TARGET_TYPE==Windows, Default" {
          disable-tunnel: ["MHLib64" ("name or relative path") "MHLib" ("name or relative path")] -> w268
          frame condition #0 (active) {
          }
          frame condition #1 {
          }
        }
        n115 = call <vilib>:"Error Cluster From Error Code.vi"("is warning? (False)"=FALSE, "show call chain? (False)"=TRUE, "error message (\"\")"="DLL not found!" ("error message (\"\")"), "error code (0)"=5000) -> ("error out"=w279:errorcluster)  [unwired: 5 in]
        n116 = call "GetDLLPath.vi"("DllName_32bit"="MHLib" ("name or relative path"), "DllName_64bit"=w268) -> ("file exists?"=w281:bool, "DLLPath"=w282:path)  [unwired: 8 in]
        n117 = global write "MH_DllPath_global.vi" "DllPath"(w282) -> ()
        n118 = Build Array (concatenate)(w307, w306) -> (w305:T8[])
        n119 = Select(t=errorcluster {"status"=FALSE, "code"=0, "source"=""} ("error IO"), s=w281, f=w279) -> (s? t:f=w286:errorcluster)
        n120 = property on="AllChannels" class="Clust (strict)"("Val(Sgnl)"=T1 {"Enable"=TRUE, "Offset"=0, "Level"=-100, "Edge"=0, "DeadTime"=1000, "UseDeadTime"=FALSE, "SetEnableAllChan"=TRUE, "SetEdgeAllChan"=TRUE, "SetLevelAllChan"=TRUE, "SetOffsetAllChan"=TRUE, "SetUseDTAllChan"=TRUE, "SetDeadTAllChan"=TRUE} ("AllChannels")) -> ()  [unwired: 2 in, 2 out]
        n121 = property on="HistoGraph" class="WFGraph (strict)"("LegPlotMin"=u32 8 ("Legend:Plot Minimum")) -> ()  [unwired: 2 in, 2 out]
        n122 = global read "MH_LibVersion_global.vi" "Library Version"() -> (w277:string)
        n123 = property on="Settings" class="Bool (strict)"("Val(Sgnl)"=TRUE ("Value (Signaling)")) -> ()  [unwired: 2 in, 2 out]
        n124 = property on="Scale" class="Bool (strict)"("Val(Sgnl)"=FALSE ("Value (Signaling)")) -> ()  [unwired: 2 in, 2 out]
        n125 = call "InitMH_UIThread.vi"("error in (no error)"=w286, "Mode"=w269, "refsource"=w278, "Library Version"=w277) -> ("error out"=w308:errorcluster, "Init Info"=w310:T5, "DevIdx"=w309:i32)  [unwired: 5 in]
        n126 = local write "SyncDivider"(w304) -> ()
        n127 = local write "SyncOffset"(w303) -> ()
        n128 = local write "SyncEdge"(w302) -> ()
        n129 = local write "SyncLevel"(w301) -> ()
        n130 = local write "UseDeadTime"(w267) -> ()
        n131 = local write "SyncDeadTime"(w266) -> ()
        n132 = local write "Binning"(w300) -> ()
        n133 = local write "HistoOffset"(w299) -> ()
        n134 = local write "HistoLength"(w297) -> ()
        n135 = local write "StopOvl."(w296) -> ()
        n136 = local write "OvlLevel"(w295) -> ()
        n137 = local write "Start"(w294) -> ()
        n138 = local write "Run continuously"(w292) -> ()
        n139 = local write "AcqTime"(w298) -> ()
        n140 = Bundle By Name(cluster=w290, "DevIdx"=w309, "Init Info"=w310, "Status"="Initialized!") -> (w289:T4)
        n141 = Unbundle By Name(w289) -> ("Init Info.Bin Steps"=w288:i32, "Init Info.Base Resolution"=w259:dbl, "Init Info.nchannels"=w264:i32)
        n142 = Initialize Array(u32 0, w264, 1024 ("dimension size")) -> (w271:u32[][])
        n143 = call "MH_InitChannels.vi"("nchannels"=w264) -> ("SetInpChan"=w262:T6[], "Channels"=w263:T3[])  [unwired: 9 in]
        n144 = To Unsigned Long Integer(number=w259) -> (unsigned 32bit integer=w260:u32)
        n145 = Divide(x=w259, y=1000.0) -> (x/y=w272:dbl)
        n146 = property on="Offset" class="DigNum (strict)"("Increment"=w259) -> ()  [unwired: 2 in, 2 out]
        n147 = property on="SyncOffset" class="DigNum (strict)"("Increment"=w259) -> ()  [unwired: 2 in, 2 out]
        n148 = property on="Offset" class="DigNum (strict)"("Increment"=w259) -> ()  [unwired: 2 in, 2 out]
        n149 = call "MH_CalcBinningValues.vi"("BaseResolution"=w260, "Bin Steps"=w288) -> ("BinningValues"=w293:cluster{"String":string, "Value":i32}[])  [unwired: 9 in]
        n150 = Bundle(0.0, w272, w271) -> (w265:cluster{dbl, dbl, u32[][]})  [unwired: 1 in]
        n151 = for {
          N: w264 -> [_]
          tunnel: w265 -> [w313]
          i -> [w315]
          n152 = Increment(x=w315) -> (x+1=w314:i32)
          n153 = Format Into String(format string="Ch.%d", w314) -> (resulting string=w316:string)  [unwired: 2 in, 1 out]
          n154 = property on="HistoGraph" class="WFGraph (strict)"("Value"=w313, "Active Plot"=w315, "Plot.Plot Name"=w316) -> ()  [unwired: 2 in, 2 out]
        }
        n155 = property on="Binning" class="Ring (strict)"("StringsAndValues[]"=w293) -> ()  [unwired: 2 in, 2 out]
        n156 = local write "Channels"(w263) -> ()
        n157 = Bundle By Name(cluster=w289, "Channels"=w263, "SetInpChan"=w262, "SyncDivider"=w304, "SyncOffset"=w303, "SyncEdge"=w302, "SyncLevel"=w301, "UseDeadTime"=w267, "SyncDeadTime"=w266, "Binning"=w300, "HistoOffset"=w299, "AcqTime"=w298, "HistoLen"=w297, "StopOvl."=w296, "OvlLevel"=w295, "StartMeas"=w294, "Run cont."=w292) -> (w285:T4)
      }
      frame "SetInpChan" {
        n158 = Unbundle By Name(w325) -> ("DevIdx"=w320:i32, "Init Info.features"=w318:i32, "SetInpChan"=w323:T6[], "Channels"=w319:T3[])
        n159 = for {
          tunnel: w319 -> [w330]
          tunnel: w323 -> [w334] mode=indexing
          shift-right: [w332] -> w322
          shift-left: errorcluster {"status"=FALSE, "code"=0, "source"=""} ("error out") -> [w331]
          tunnel: w320 -> [w328]
          tunnel: w318 -> [w326]
          n160 = Unbundle By Name(w334) -> ("Cmds"=w333:T7[], "Channel"=w327:i32)
          n161 = Index Array(array=w330, index=w327) -> (element=w329:T3)
          n162 = for {
            tunnel: w333 -> [w341] mode=indexing
            tunnel: w327 -> [w340]
            shift-right: [w339] -> w332
            shift-left: w331 -> [w338]
            tunnel: w329 -> [w337]
            tunnel: w328 -> [w336]
            tunnel: w326 -> [w335]
            n163 = case shown="\"SetInpChanOffset\"" w341 {
              tunnel: w340 -> [_ w347 w354 w359 w375]
              tunnel: [w342 w346 w353 w363 w380] -> w339
              tunnel: w338 -> [w342 w345 w352 w362 w379]
              tunnel: w337 -> [_ w344 w351 w361 w378]
              tunnel: w336 -> [_ w343 w350 w360 w377]
              tunnel: w335 -> [_ _ _ w356 _]
              frame Default {
              }
              frame "SetInpChanEnable" {
                n164 = Unbundle By Name(w344) -> ("Enable"=w348:bool)
                n165 = call "MH_SetInputChannelEnable.vi"("error in (no error)"=w345, "enable"=w348, "channel"=w347, "devidx"=w343) -> ("error out"=w346:errorcluster)  [unwired: 6 in, 1 out]
              }
              frame "SetInpChanOffset" {
                n166 = Unbundle By Name(w351) -> ("Offset"=w349:i32)
                n167 = call "MH_SetInputChannelOffset.vi"("error in (no error)"=w352, "Offset"=w349, "channel"=w354, "devidx"=w350) -> ("error out"=w353:errorcluster)  [unwired: 6 in, 1 out]
              }
              frame "SetInpChanDeadTime" {
                w357 = 32  # FEATURE_PROG_TD
                n168 = And(x=w356, y=w357) -> (x .and. y?=w358:i32)
                n169 = Not Equal To 0?(x=w358) -> (x != 0?=w355:bool)
                n170 = case shown="False" w355 {
                  tunnel: [w364 w373] -> w363
                  tunnel: w362 -> [w364 w372]
                  tunnel: w361 -> [_ w371]
                  tunnel: w360 -> [_ w370]
                  tunnel: w359 -> [_ w368]
                  frame False {
                  }
                  frame True {
                    n171 = Unbundle By Name(w371) -> ("UseDeadTime"=w367:bool, "DeadTime"=w369:i32)
                    n172 = Boolean To (0,1)(Boolean=w367) -> (0, 1=w366:i16)
                    n173 = To Long Integer(number=w366) -> (32bit integer=w365:i32)
                    n174 = call "MH_SetInputDeadTime.vi"("channel"=w368, "error in (no error)"=w372, "deadtime"=w369, "on"=w365, "devidx"=w370) -> ("error out"=w373:errorcluster)  [unwired: 5 in, 1 out]
                  }
                }
              }
              frame "SetInpChanTrg" {
                n175 = Unbundle By Name(w378) -> ("Level"=w374:i32, "Edge"=w376:i32)
                n176 = call "MH_SetInputEdgeTrg.vi"("channel"=w375, "error in (no error)"=w379, "edge"=w376, "level"=w374, "devidx"=w377) -> ("error out"=w380:errorcluster)  [unwired: 5 in, 1 out]
              }
            }
          }
        }
      }
      frame "SetSyncDivider" {
        n177 = Unbundle By Name(w388) -> ("DevIdx"=w387:i32, "SyncDivider"=w383:i32)
        n178 = Power Of 2(x=w383) -> (2^x=w382:dbl)
        n179 = To Long Integer(number=w382) -> (32bit integer=w381:i32)
        n180 = call "MH_SetSyncDiv.vi"("SyncDivider"=w381, "devidx"=w387) -> ("error out"=w385:errorcluster)  [unwired: 8 in, 1 out]
        n181 = flat-sequence {
          tunnel: w385 -> [w389]
          tunnel: [w389] -> w384
          frame #0 {
            n182 = Wait (ms)(milliseconds to wait=u32 100) -> ()  [unwired: 1 out]
          }
        }
      }
      frame "SetSyncTrg" {
        n183 = Unbundle By Name(w396) -> ("DevIdx"=w393:i32, "SyncLevel"=w391:i32, "SyncEdge"=w392:i32)
        n184 = call "MH_SetSyncEdgeTrg.vi"("edge"=w392, "level"=w391, "devidx"=w393) -> ("error out"=w394:errorcluster)  [unwired: 7 in, 1 out]
      }
      frame "SetSyncDeadTime" {
        w399 = 32  # FEATURE_PROG_TD
        n185 = Unbundle By Name(w408) -> ("DevIdx"=w405:i32, "UseDeadTime"=w403:bool, "SyncDeadTime"=w404:i32, "Init Info.features"=w398:i32)
        n186 = Boolean To (0,1)(Boolean=w403) -> (0, 1=w402:i16)
        n187 = And(x=w398, y=w399) -> (x .and. y?=w400:i32)
        n188 = To Long Integer(number=w402) -> (32bit integer=w401:i32)
        n189 = Not Equal To 0?(x=w400) -> (x != 0?=w397:bool)
        n190 = case shown="False" w397 {
          tunnel: [_ w412] -> w406
          tunnel: w405 -> [_ w411]
          tunnel: w404 -> [_ w410]
          tunnel: w401 -> [_ w409]
          frame False {
          }
          frame True {
            n191 = call "MH_SetSyncDeadTime.vi"("deadtime"=w410, "on"=w409, "devidx"=w411) -> ("error out"=w412:errorcluster)  [unwired: 7 in, 1 out]
          }
        }
      }
      frame "SetSyncOffset" {
        n192 = Unbundle By Name(w417) -> ("DevIdx"=w415:i32, "SyncOffset"=w414:i32)
        n193 = call "MH_SetSyncChannelOffset.vi"("Offset"=w414, "devidx"=w415) -> ("error out"=w416:errorcluster)  [unwired: 8 in, 1 out]
      }
      frame "SetBinning" {
        # "When binning is changed the new resolution is querried"
        n194 = Unbundle By Name(w424) -> ("DevIdx"=w422:i32, "Binning"=w421:i32)
        n195 = call "MH_SetBinning.vi"("Binning"=w421, "devidx"=w422) -> ("error out"=w423:errorcluster)  [unwired: 8 in, 1 out]
        n196 = Build Array (concatenate)(MH_UIThread_Cmds."GetResolution", w419) -> (w420:T8[])
      }
      frame "SetHistoOffset" {
        n197 = Unbundle By Name(w429) -> ("DevIdx"=w426:i32, "HistoOffset"=w425:i32)
        n198 = call "MH_SetOffset.vi"("Offset"=w425, "devidx"=w426) -> ("error out"=w427:errorcluster)  [unwired: 8 in, 1 out]
      }
      frame "SetHistoLen" {
        n199 = Unbundle By Name(w432) -> ("DevIdx"=w434:i32, "HistoLen"=w433:i32)
        n200 = call "MH_SetHistoLen.vi"("lencode"=w433, "devidx"=w434) -> ("error out"=w435:errorcluster, "actuallen"=w430:i32)  [unwired: 7 in, 1 out]
        n201 = Bundle By Name(cluster=w432, "HistoLength"=w430) -> (w431:T4)
      }
      frame "SetStopOvl" {
        n202 = Unbundle By Name(w442) -> ("DevIdx"=w439:i32, "StopOvl."=w438:bool, "OvlLevel"=w437:u32)
        n203 = call "MH_SetStopOverflow.vi"("stopcount"=w437, "StopOnOverflow"=w438, "devidx"=w439) -> ("error out"=w440:errorcluster)  [unwired: 7 in, 1 out]
      }
      frame "GetAllRates" {
        # "An alternative to GetRates"
        n204 = Unbundle By Name(w451) -> ("DevIdx"=w448:i32, "Init Info.nchannels"=w443:i32)
        n205 = call "MH_AllocateCntRateBuffer.vi"("NumChan"=w443) -> ("Buffer"=w444:i32[])  [unwired: 10 in]
        n206 = call "MH_GetAllCountRates.vi"("cntrates_buf"=w444, "devidx"=w448) -> ("error out"=w445:errorcluster, "cntrates"=→"CountRates":i32[], "syncrate"=w447:i32)  [unwired: 6 in, 1 out]
        n207 = Format Into String(format string="Sync Rate: %d cps\n", w447) -> (resulting string=→"SyncRate":string)  [unwired: 2 in, 1 out]
      }
      frame "GetRates" {
        # "An alternative to GetAllRates"
        n208 = Unbundle By Name(w462) -> ("Init Info.nchannels"=w457:i32, "Channels"=w459:T3[], "DevIdx"=w458:i32)
        n209 = call "MH_GetSyncRate.vi"("devidx"=w458) -> ("error out"=w455:errorcluster, "syncrate"=w454:i32)  [unwired: 8 in, 1 out]
        n210 = Format Into String(format string="Sync Rate: %d cps\n", w454) -> (resulting string=w456:string)  [unwired: 2 in, 1 out]
        n211 = for {
          N: w457 -> [_]
          tunnel: w458 -> [w469]
          tunnel: [w466] -> w453 mode=indexing
          shift-right: [w468] -> w461
          shift-left: w455 -> [w470]
          tunnel: w459 -> [w465] mode=indexing
          i -> [w467]
          n212 = Unbundle By Name(w465) -> ("Enable"=w464:bool)
          n213 = case shown="True" w464 {
            tunnel: w470 -> [w471 w476]
            tunnel: w469 -> [_ w475]
            tunnel: [w471 w474] -> w468
            tunnel: w467 -> [_ w473]
            tunnel: [_ w472] -> w466
            frame False {
            }
            frame True {
              n214 = call "MH_GetCountRate.vi"("error in (no error)"=w476, "Channel"=w473, "devidx"=w475) -> ("error out"=w474:errorcluster, "rate"=w472:i32)  [unwired: 6 in, 1 out]
            }
          }
        }
        n215 = local write "SyncRate"(w456) -> ()
        n216 = local write "CountRates"(w453) -> ()
      }
      frame "StartMeas" {
        n217 = Unbundle By Name(w484) -> ("AcqTime"=w480:i32, "DevIdx"=w481:i32)
        n218 = call "MH_ClearHistMem.vi"("devidx"=w481) -> ("error out"=w482:errorcluster)  [unwired: 9 in, 1 out]
        n219 = call "MH_StartMeas.vi"("error in (no error)"=w482, "tacq"=w480, "devidx"=w481) -> ("error out"=w483:errorcluster)  [unwired: 7 in, 1 out]
        n220 = Build Array (concatenate)(w479, MH_UIThread_Cmds."GetAllHistos") -> (w478:T8[])
      }
      frame "StopMeas" {
        n221 = Unbundle By Name(w490) -> ("Run cont."=w485:bool, "DevIdx"=w491:i32)
        n222 = call "MH_StopMeas.vi"("devidx"=w491) -> ("error out"=w492:errorcluster)  [unwired: 9 in, 1 out]
        n223 = case shown="False" w485 {
          tunnel: w490 -> [w496 w498]
          tunnel: [w495 w498] -> w489
          tunnel: [w493 w497] -> w488
          frame False {
            w493 = T8[] [enum."GetAllHistos"] items=["Idle", "Init", "SetInpChan", "SetSyncDivider", "SetSyncTrg", "SetSyncOffset", "SetSyncDeadTime", "SetBinning", "SetHistoOffset", "SetHistoLen", "SetStopOvl", "SetBitShift", "SetHistoAcqTime", "GetRates", "GetAllRates", "StartMeas", "StopMeas", "AbortMeas", "GetResolution", "GetHistos", "GetAllHistos", "ReadFiFo", "WriteStatus", "Resize", "EnableControls", "DisableControls", "Error", "Exit"]
            w494 = FALSE ("StartMeas")
            n224 = Bundle By Name(cluster=w496, "StartMeas"=w494) -> (w495:T4)
            n225 = local write "Start"(w494) -> ()
          }
          frame True {
            w497 = T8[] [enum."GetAllHistos", enum."StartMeas"] items=["Idle", "Init", "SetInpChan", "SetSyncDivider", "SetSyncTrg", "SetSyncOffset", "SetSyncDeadTime", "SetBinning", "SetHistoOffset", "SetHistoLen", "SetStopOvl", "SetBitShift", "SetHistoAcqTime", "GetRates", "GetAllRates", "StartMeas", "StopMeas", "AbortMeas", "GetResolution", "GetHistos", "GetAllHistos", "ReadFiFo", "WriteStatus", "Resize", "EnableControls", "DisableControls", "Error", "Exit"]
          }
        }
        n226 = Build Array (concatenate)(w487, w488) -> (w486:T8[])
      }
      frame "AbortMeas" {
        w502 = T8[] [enum."GetAllHistos"] items=["Idle", "Init", "SetInpChan", "SetSyncDivider", "SetSyncTrg", "SetSyncOffset", "SetSyncDeadTime", "SetBinning", "SetHistoOffset", "SetHistoLen", "SetStopOvl", "SetBitShift", "SetHistoAcqTime", "GetRates", "GetAllRates", "StartMeas", "StopMeas", "AbortMeas", "GetResolution", "GetHistos", "GetAllHistos", "ReadFiFo", "WriteStatus", "Resize", "EnableControls", "DisableControls", "Error", "Exit"]
        w499 = FALSE ("StartMeas")
        n227 = Unbundle By Name(w504) -> ("DevIdx"=w505:i32)
        n228 = call "MH_StopMeas.vi"("devidx"=w505) -> ("error out"=w506:errorcluster)  [unwired: 9 in, 1 out]
        n229 = Bundle By Name(cluster=w504, "StartMeas"=w499) -> (w503:T4)
        n230 = local write "Start"(w499) -> ()
        n231 = Build Array (concatenate)(w501, w502) -> (w500:T8[])
      }
      frame "GetResolution" {
        # "Resolution in ns"
        # "Gets resolution in ps"
        # "Resolution is saved in UIThread Data cluster in ns"
        n232 = Unbundle By Name(w511) -> ("DevIdx"=w513:i32)
        n233 = call "MH_GetResolution.vi"("devidx"=w513) -> ("error out"=w512:errorcluster, "resolution"=w509:dbl)  [unwired: 8 in, 1 out]
        n234 = Divide(x=w509, y=1000.0) -> (x/y=w507:dbl)
        n235 = Bundle By Name(cluster=w511, "Resolution"=w507) -> (w510:T4)
      }
      frame "GetAllHistos" {
        w527 = 1  # FLAG_OVERFLOW
        # "Provides a buffer (U32-array of length 'HistoLength' x nchannels) for all histograms."
        # "An alternative to GetHistos"
        n236 = Unbundle By Name(w538) -> ("Resolution"=w537:dbl, "DevIdx"=w517:i32, "HistoLength"=w520:i32, "Init Info.nchannels"=w521:i32)
        n237 = call "MH_AllocateAllHistoBuffer.vi"("NumChan"=w521, "HistoLength"=w520) -> ("Buffer"=w518:u32[])  [unwired: 9 in]
        n238 = call "MH_GetAllHistograms.vi"("Chcount"=w518, "devidx"=w517) -> ("error out"=w515:errorcluster, "Histograms"=w516:u32[])  [unwired: 7 in, 1 out]
        n239 = Reshape Array(w516, w521, w520) -> (w519:u32[][])
        n240 = for {
          tunnel: [w540] -> w529 mode=indexing
          shift-right: [w542] -> w523
          shift-left: "Total Counts:\t\t" -> [w541]
          tunnel: w519 -> [w540] mode=indexing
          i -> [w546]
          n241 = Add Array Elements(numeric array=w540) -> (sum=w543:u32)
          n242 = Increment(x=w546) -> (x+1=w544:i32)
          n243 = Format Into String(format string="Ch.%2d: %d cnts.\t\t", initial string=w541, w544, w543) -> (resulting string=w542:string)  [unwired: 1 in, 1 out]
        }
        n244 = call "CalcRate.vi"("Refresh(ms)"=u32 500) -> ("Rate / Hz"=w535:dbl)  [unwired: 8 in, 2 out]
        n245 = Format Into String(format string="Readout Rate: %.1f Hz\\t\\t", w535) -> (resulting string=w533:string)  [unwired: 2 in, 1 out]
        n246 = Concatenate Strings(w533, w523) -> (w532:string)
        n247 = Bundle(0.0, "Resolution"=w537, "Histograms"=w529) -> (→"HistoGraph":T13)  [unwired: 1 in]
        n248 = local write "Status"(w532) -> ()
        n249 = call "MH_GetFlags.vi"("error in (no error)"=w515) -> ("error out"=w536:errorcluster, "flags"=w526:i32)  [unwired: 8 in, 1 out]
        n250 = And(x=w527, y=w526) -> (x .and. y?=w528:i32)
        n251 = Not Equal To 0?(x=w528) -> (x != 0?=→"OverFlow":bool)
      }
      frame "GetHistos" {
        w556 = 1  # FLAG_OVERFLOW
        # "Provides a buffer (U32-array of length 'HistoLength') for histograms."
        # "An alternative to GetAllHistos"
        n252 = Unbundle By Name(w570) -> ("Resolution"=w567:dbl, "Init Info.nchannels"=w549:i32, "Channels"=w550:T3[], "DevIdx"=w569:i32, "HistoLength"=w568:i32)
        n253 = call "MH_AllocateHistoBuffer.vi"("HistoLength"=w568) -> ("Buffer"=w561:u32[])  [unwired: 10 in]
        n254 = for {
          N: w549 -> [_]
          tunnel: w569 -> [w584]
          tunnel: [w572] -> w559 mode=indexing
          tunnel: w561 -> [w582]
          shift-right: [w583] -> w558
          shift-left: errorcluster {"status"=FALSE, "code"=0, "source"=""} ("error IO") -> [w576]
          shift-right: [w577] -> w552
          shift-left: "Total Counts:\t\t" -> [w575]
          tunnel: w550 -> [w574] mode=indexing
          i -> [w581]
          n255 = Unbundle By Name(w574) -> ("Enable"=w573:bool)
          n256 = case shown="True" w573 {
            tunnel: w584 -> [_ w592]
            tunnel: [w585 w591] -> w583
            tunnel: w582 -> [w586 w590]
            tunnel: [w586 w589] -> w572
            tunnel: w581 -> [_ w588]
            tunnel: w576 -> [w585 w587]
            frame False {
            }
            frame True {
              n257 = call "MH_GetHistogram.vi"("Chcount"=w590, "error in (no error)"=w587, "channel"=w588, "devidx"=w592) -> ("error out"=w591:errorcluster, "Histogram"=w589:u32[])  [unwired: 5 in, 1 out]
            }
          }
          n258 = Add Array Elements(numeric array=w572) -> (sum=w578:u32)
          n259 = Increment(x=w581) -> (x+1=w579:i32)
          n260 = Format Into String(format string="Ch.%2d: %d cnts.\t\t", initial string=w575, w579, w578) -> (resulting string=w577:string)  [unwired: 1 in, 1 out]
        }
        n261 = call "CalcRate.vi"("Refresh(ms)"=u32 500) -> ("Rate / Hz"=w565:dbl)  [unwired: 8 in, 2 out]
        n262 = Format Into String(format string="Readout Rate: %.1f Hz\\t\\t", w565) -> (resulting string=w563:string)  [unwired: 2 in, 1 out]
        n263 = Concatenate Strings(w563, w552) -> (w562:string)
        n264 = Bundle(0.0, "Resolution"=w567, "Histogram"=w559) -> (w547:T2)  [unwired: 1 in]
        n265 = local write "HistoGraph"(w547) -> ()
        n266 = local write "Status"(w562) -> ()
        n267 = call "MH_GetFlags.vi"("error in (no error)"=w558) -> ("error out"=w566:errorcluster, "flags"=w555:i32)  [unwired: 8 in, 1 out]
        n268 = And(x=w556, y=w555) -> (x .and. y?=w557:i32)
        n269 = Not Equal To 0?(x=w557) -> (x != 0?=w548:bool)
        n270 = local write "OverFlow"(w548) -> ()
      }
      frame "WriteStatus" {
        n271 = Unbundle By Name(w594) -> ("Status"=→"Status":string)
      }
      frame "Resize" {
        n272 = property on="Pane 3" class="Pane"() -> ("Width"=w601:u32)  [unwired: 2 in, 2 out]
        n273 = Subtract(x=w601, y=i16 100 ("b")) -> (x-y=w607:u32)
        n274 = Unbundle By Name(w596) -> ("Init Info.nchannels"=w604:i32)
        n275 = Quotient & Remainder(x=w607, y=i16 99 ("m")) -> (floor(x/y)=w606:u32)  [unwired: 1 out]
        n276 = In Range and Coerce(upper limit=w604, x=w606, lower limit=4) -> (coerced(x)=w605:u32)  [unwired: 1 out]
        n277 = Equal?(x=w604, y=w605) -> (x = y?=w603:bool)
        n278 = Not(x=w603) -> (.not. x?=w602:bool)
        n279 = property on="Channels" class="Arr (strict)"("HorizScroll"=w602, "Number of Columns"=w605, "Index Values"=u32[] [0]) -> ()  [unwired: 2 in, 2 out]
      }
      frame "EnableControls" {
        n280 = property class="VI"() -> ("Panel"=w612:refnum<vi>)  [unwired: 2 in, 2 out]
        n281 = property class="Pnl"(reference=w612) -> ("Controls[]"=w611:refnum<vi>[])  [unwired: 1 in, 2 out]
        n282 = property class="Pnl"(reference=w612) -> ("Decos[]"=w613:refnum<vi>[])  [unwired: 1 in, 2 out]
        n283 = for {
          tunnel: w613 -> [w617] mode=indexing
          tunnel: TRUE -> [w616]
          n284 = property class="Decor"(reference=w617, "Visible"=w616) -> ()  [unwired: 1 in, 2 out]
        }
        n285 = for {
          tunnel: w611 -> [w620] mode=indexing
          tunnel: T9."Enabled" ("Disabled") -> [w619]
          tunnel: [w618] -> _
          n286 = property class="Ctl"(reference=w620, "DisabledEnum"=w619) -> (error out=w618:errorcluster)  [unwired: 1 in, 1 out]
        }
      }
      frame "DisableControls" {
        n287 = property class="VI"() -> ("Panel"=w624:refnum<vi>)  [unwired: 2 in, 2 out]
        n288 = property class="Pnl"(reference=w624) -> ("Controls[]"=w623:refnum<vi>[])  [unwired: 1 in, 2 out]
        n289 = property class="Pnl"(reference=w624) -> ("Decos[]"=w625:refnum<vi>[])  [unwired: 1 in, 2 out]
        n290 = for {
          tunnel: w625 -> [w629] mode=indexing
          tunnel: FALSE -> [w628]
          n291 = property class="Decor"(reference=w629, "Visible"=w628) -> ()  [unwired: 1 in, 2 out]
        }
        n292 = for {
          tunnel: w623 -> [w632] mode=indexing
          tunnel: T9."Disabled and Grayed Out" ("Disabled") -> [w631]
          tunnel: [w630] -> _
          n293 = property class="Ctl"(reference=w632, "DisabledEnum"=w631) -> (error out=w630:errorcluster)  [unwired: 1 in, 1 out]
        }
      }
      frame "Error" {
        w633 = T8[] [enum."Exit"] items=["Idle", "Init", "SetInpChan", "SetSyncDivider", "SetSyncTrg", "SetSyncOffset", "SetSyncDeadTime", "SetBinning", "SetHistoOffset", "SetHistoLen", "SetStopOvl", "SetBitShift", "SetHistoAcqTime", "GetRates", "GetAllRates", "StartMeas", "StopMeas", "AbortMeas", "GetResolution", "GetHistos", "GetAllHistos", "ReadFiFo", "WriteStatus", "Resize", "EnableControls", "DisableControls", "Error", "Exit"]
        w636 = T14 1 items=["no dialog", "OK message", "continue or stop message", "OK message + warnings", "continue/stop + warnings"] ("type of dialog (OK msg:1)")
        # "Error case: If an error occures the user is informed and the programm terminates. Add your own code to handle error events (e.g. exception lists, etc.)"
        n294 = call <vilib>:"Simple Error Handler.vi"("type of dialog (OK msg:1)"=w636, "error in (no error)"=w635) -> ()  [unwired: 3 in, 5 out]
      }
      frame "Exit" {
        n295 = Unbundle By Name(w640) -> ("DevIdx"=w639:i32)
        n296 = call "MH_CloseDevice.vi"("devidx"=w639) -> ("error out"=w638:errorcluster)  [unwired: 9 in, 1 out]
      }
    }
    n297 = call "MH_EnQError.vi"("error in (no error)"=w8, "Cmds_in"=w6) -> ("error out"=w7:errorcluster, "Cmds_out"=w5:T8[])  [unwired: 8 in]
  }
